vi "parseSetTemporaryAddressError.vi"(8 "error in (no error)":errorcluster, 10 "DynamicFrameParser":refnum<class "DynamicFrameParser.lvclass">, 11 "ILC in":refnum<class "ILC.lvclass">) -> (0 "error out":errorcluster, 3 "ILC out":refnum<class "ILC.lvclass">)   [LabVIEW 2016, in "RTILC.lvlib" / "ILC.lvclass"]
uses:
  ILC.lvclass
  Common_RT_Modbus/DynamicFrameParser/DynamicFrameParser.lvclass
  ILC.lvclass/ILC.ctl
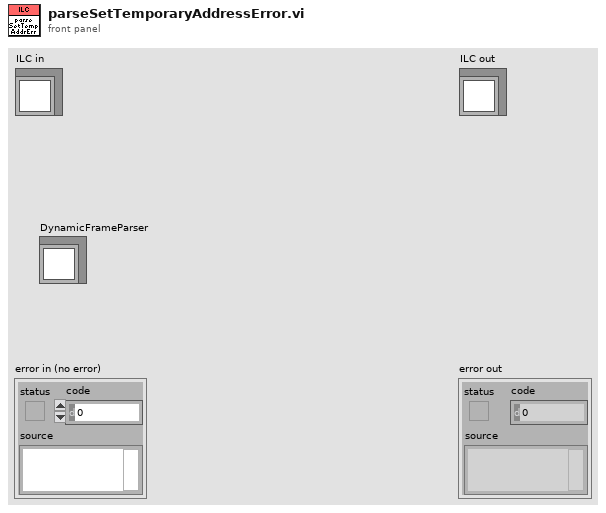
[diagram p1: front panel]
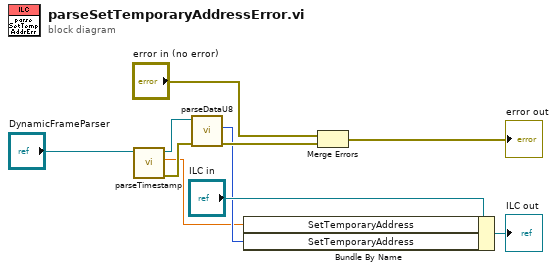
[diagram p0: block diagram]
diagram:
  n1 = call "parseTimestamp.vi"("FrameParser in"="DynamicFrameParser") -> ("error out"=w2:errorcluster, "Timestamp"=w1:dbl, "FrameParser out"=w3:refnum<class "DynamicFrameParser.lvclass">)  [unwired: 8 in]
  n2 = call "parseDataU8.vi"("error in (no error)"=w2, "FrameParser in"=w3) -> ("error out"=w6:errorcluster, "Data"=w5:u8)  [unwired: 7 in, 1 out]
  n3 = Bundle By Name(cluster="ILC in", "SetTemporaryAddress"=w1, "SetTemporaryAddress"=w5) -> (→"ILC out":refnum<class "ILC.lvclass">)
  n4 = Merge Errors("error in (no error)", w6) -> (→"error out":errorcluster)
